vi "Write Attribute Values.vi"(10 "Attribute Values":variant[](array[variant]), 11 "Sequence Dialog in":refnum<class "TestStep Edit Dialog.lvclass">) -> (3 "Sequence Dialog out":refnum<class "TestStep Edit Dialog.lvclass">)   [LabVIEW 2017, in "TestStep Edit Dialog.lvclass"]
uses:
  TestStep Edit Dialog.lvclass
  TestStep Edit Dialog.lvclass/TestStep Edit Dialog.ctl
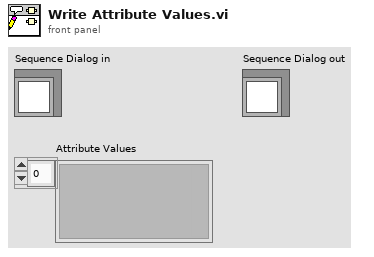
[diagram p1: front panel]
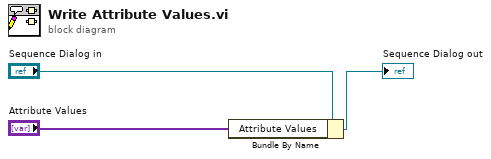
[diagram p0: block diagram]
diagram:
  n1 = Bundle By Name(cluster="Sequence Dialog in", "Attribute Values"="Attribute Values") -> (→"Sequence Dialog out":refnum<class "TestStep Edit Dialog.lvclass">)
